vi "Inverse Time Curves.vi"   [LabVIEW 2012, in "NI_EP_Protection.lvlib"]
doc: "Generates memory initial values and memory size, which contain the information of the inverse time curves, for the FPGA Inverse Time Delay VI to use. You can compensate for the processing delay of the input energizing quantity under a specific G/Gs to achieve higher operate time accuracy."
uses:
  <vilib>/addons/Electrical Power/Protection/NI_EP_Protection.lvlib
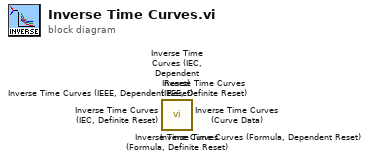
[diagram p0: block diagram]
diagram:
  n1 = call <vilib>:"Inverse Time Curves (Formula, Definite Reset).vi"() -> ()  [unwired: 8 in, 4 out]
  n2 = call <vilib>:"Inverse Time Curves (IEEE, Definite Reset).vi"() -> ()  [unwired: 8 in, 4 out]
  n3 = call <vilib>:"Inverse Time Curves (IEC, Definite Reset).vi"() -> ()  [unwired: 8 in, 4 out]
  n4 = call <vilib>:"Inverse Time Curves (Curve Data).vi"() -> ()  [unwired: 8 in, 4 out]
  n5 = call <vilib>:"Inverse Time Curves (IEEE, Dependent Reset).vi"() -> ()  [unwired: 8 in, 4 out]
  n6 = call <vilib>:"Inverse Time Curves (IEC, Dependent Reset).vi"() -> ()  [unwired: 8 in, 4 out]
  n7 = call <vilib>:"Inverse Time Curves (Formula, Dependent Reset).vi"() -> ()  [unwired: 8 in, 4 out]
